vi "FTW-VIServer-VI-Metadata.vi"(0 "VI Filepath":path, 11 "error in":errorcluster) -> (4 "Front Panel Title":string, 6 "VI Description":string, 15 "error out":errorcluster)   [LabVIEW 2013]
panel:
  # "Inputs"
  # "Outputs"
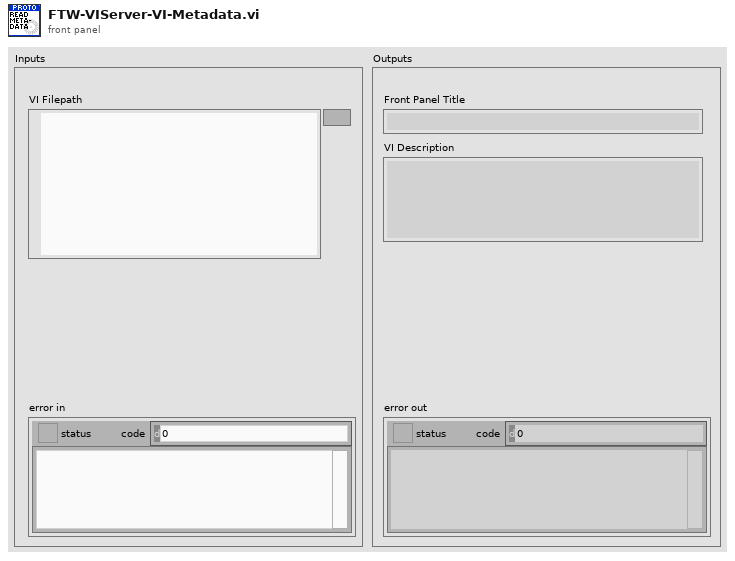
[diagram p1: front panel]
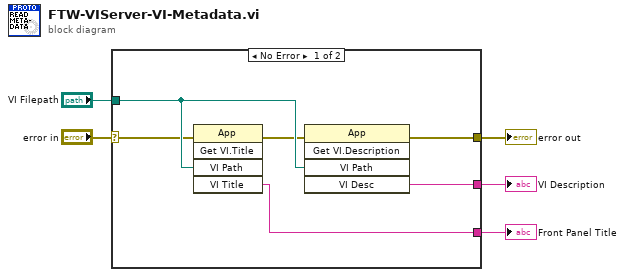
[diagram p0: block diagram]
diagram:
  n1 = case shown="No Error" "error in" {
    selector: "error in" -> [w7 w12]
    tunnel: [w6 w12] -> w5
    tunnel: [w10 _] -> w3
    tunnel: [w9 _] -> w2
    tunnel: "VI Filepath" -> [w11 _]
    frame No Error {
      n2 = invoke class="App" method="Get VI.Title"(error in=w7, "VI Path"=w11) -> (error out=w8:errorcluster, "VI Title"=w10:string)  [unwired: 3 in, 3 out]
      n3 = invoke class="App" method="Get VI.Description"(error in=w8, "VI Path"=w11) -> (error out=w6:errorcluster, "VI Desc"=w9:string)  [unwired: 3 in, 3 out]
    }
    frame Error {
    }
  }
  "error out" <- w5
  "Front Panel Title" <- w3
  "VI Description" <- w2
